vi "Find status indexes.vi"(8 "error in (no error)":errorcluster, 11 "Custom Device ref":T1 format="%.0x") -> (0 "error out":errorcluster, 2 "Indexes":i32[](array[numeric]), 3 "Custom Device ref":T1 format="%.0x")   [LabVIEW 2019, in "GE_RM_Real Time.lvlib"]
uses:
  GE_RM_Real Time.lvlib
  Custom Device Item Ref.ctl
  Custom Device Utility Library.lvlib
  Custom Device API.lvlib
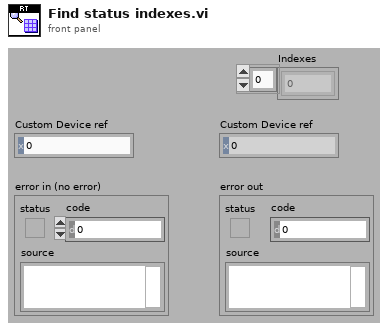
[diagram p1: front panel]
types:
  T1 = typedef "Custom Device API.lvlib/Custom Device Item Ref.ctl" = u64
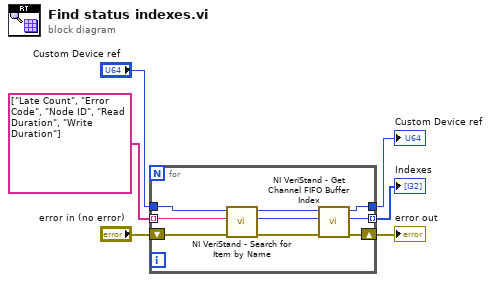
[diagram p0: block diagram]
diagram:
  n1 = for {
    tunnel: "Custom Device ref" -> [w14]
    tunnel: string[] ["Late Count", "Error Code", "Node ID", "Read Duration", "Write Duration"] -> [w13] mode=indexing
    shift-right: [w9] -> w2
    shift-left: "error in (no error)" -> [w15]
    tunnel: [w8] -> w3 mode=indexing
    tunnel: [w7] -> w1
    n2 = call "NI VeriStand - Search for Item by Name.vi"("error in"=w15, "Item Name"=w13, "Section Ref in"=w14) -> ("error out"=w12:errorcluster, "Item Ref"=w11:T1, "Section Ref out"=w10:T1)  [unwired: 5 in, 1 out]
    n3 = call "NI VeriStand - Get Channel FIFO Buffer Index.vi"("error in"=w12, "Channel Ref"=w11, "Device Ref in"=w10) -> ("error out"=w9:errorcluster, "Channel FIFO Buffer Index"=w8:i32, "Device Ref out"=w7:T1)  [unwired: 4 in, 2 out]
  }
  "Custom Device ref" <- w1
  "error out" <- w2
  "Indexes" <- w3
